vi "RT Config - Single RT Sweep.vi"(8 "error in (no error)":errorcluster, 11 "1553 Unit Test in":refnum<class "Remote Terminal.lvclass">) -> (0 "error out":errorcluster, 3 "1553 Unit Test out":refnum<class "Remote Terminal.lvclass">)   [LabVIEW 2020, in "Unit Tests.lvlib" / "Remote Terminal.lvclass"]
uses:
  Remote Terminal.lvclass
  Remote Terminal.lvclass/Remote Terminal.ctl
  Remote Terminal/TypeDefs/RT Command Config.ctl
  Frames & Messages/TypeDefs/Command Type.ctl
  Frames & Messages/TypeDefs/Command SubAddress.ctl
  Frames & Messages/TypeDefs/Command Word Count.ctl
  Frames & Messages/TypeDefs/Simplified Parameter Data Table.ctl
  Frames & Messages/TypeDefs/Scaling Information.ctl
  Remote Terminal/TypeDefs/RT Configuration.ctl
  Remote Terminal/TypeDefs/RT-RT Timeout.ctl
  Remote Terminal/TypeDefs/Mode Code 17 Sync Configuration.ctl
  Remote Terminal/TypeDefs/RT Timetag Configuration.ctl
  Remote Terminal/Remote Terminal.lvclass
  C:/Users/MattJ/Desktop/git/bci-1553-labview-api/src/1553 SubComponent/1553 SubComponent.lvclass
  1553 Session/1553 Session.lvclass
  1553 Component/1553 Component.lvclass
  <vilib>/addons/_JKI Toolkits/Caraya/classes/Test/Test.lvclass
  BCI-1553 API.lvlib
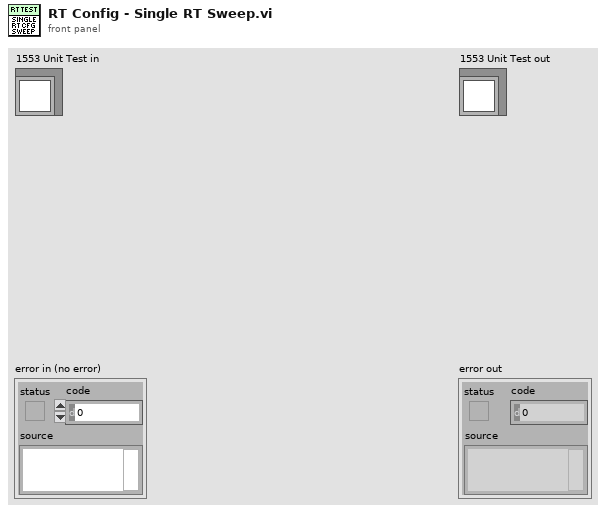
[diagram p1: front panel]
types:
  T1 = typedef "BCI-1553 API.lvlib/Simplified Parameter Data Table.ctl" = cluster{"Parameter Name":string, "Base Word":u16, "Scaling Info":T2}
  T2 = typedef "BCI-1553 API.lvlib/Scaling Information.ctl" = cluster{"Bit Offset":i32, "Bit Count":i32, "LSB Resolution":dbl, "2's Complement":bool, "Big Endian":bool, "Sign Bit":bool}
  T3 = typedef "BCI-1553 API.lvlib/Command SubAddress.ctl" = enum16{"Mode Code", "1", "2", "3", "4", "5", "6", "7", "8", "9", "10", "11", "12", "13", "14", "15", "16", "17", "18", "19", "20", "21", "22", "23", "24", "25", "26", "27", "28", "29", "30"}
  T4 = typedef "BCI-1553 API.lvlib/Command Type.ctl" = enum16{"Transmit", "Receive"}
  T5 = typedef "BCI-1553 API.lvlib/Remote Terminal.lvclass/RT Command Config.ctl" = cluster{"Command Type":T4, "SubAddress":T3, "Word Count\\Mode Code":T6, "Initial Data":u16[], "Data Fields":T1[]}
  T6 = typedef "BCI-1553 API.lvlib/Command Word Count.ctl" = enum16{"1", "2", "3", "4", "5", "6", "7", "8", "9", "10", "11", "12", "13", "14", "15", "16", "17", "18", "19", "20", "21", "22", "23", "24", "25", "26", "27", "28", "29", "30", "31", "32"}
  T7 = typedef "BCI-1553 API.lvlib/Remote Terminal.lvclass/RT Configuration.ctl" = cluster{"RT-RT Timeout":T8, "Inhibit Bus A":bool, "Inhibit Bus B":bool, "Broadcast CMD Invalid":bool, "UnDef MCs Invalid":bool, "Notice 2 Data Storage":bool, "SMCP":bool, "Temp RX Buffer":bool, "Alt BIT Enable":bool, "Auto Bus Shutdown":bool, "MC 16 SR Reset":bool, "MC 17 Sync":T9, "MC 8 Reset":bool, "Remote Terminal Timetag Config":T10}
  T8 = typedef "BCI-1553 API.lvlib/Remote Terminal.lvclass/RT-RT Timeout.ctl" = enum16{"57us", "62us", "100us", "180us"}
  T9 = typedef "BCI-1553 API.lvlib/Remote Terminal.lvclass/Mode Code 17 Sync Configuration.ctl" = enum16{"Sync if Bit 0 = 1", "Sync if Bit 0 = 0", "Sync Unconditionally"}
  T10 = typedef "BCI-1553 API.lvlib/Remote Terminal.lvclass/RT Timetag Configuration.ctl" = enum16{"Disabled", "2us", "4us", "8us", "16us", "32us", "64us"}
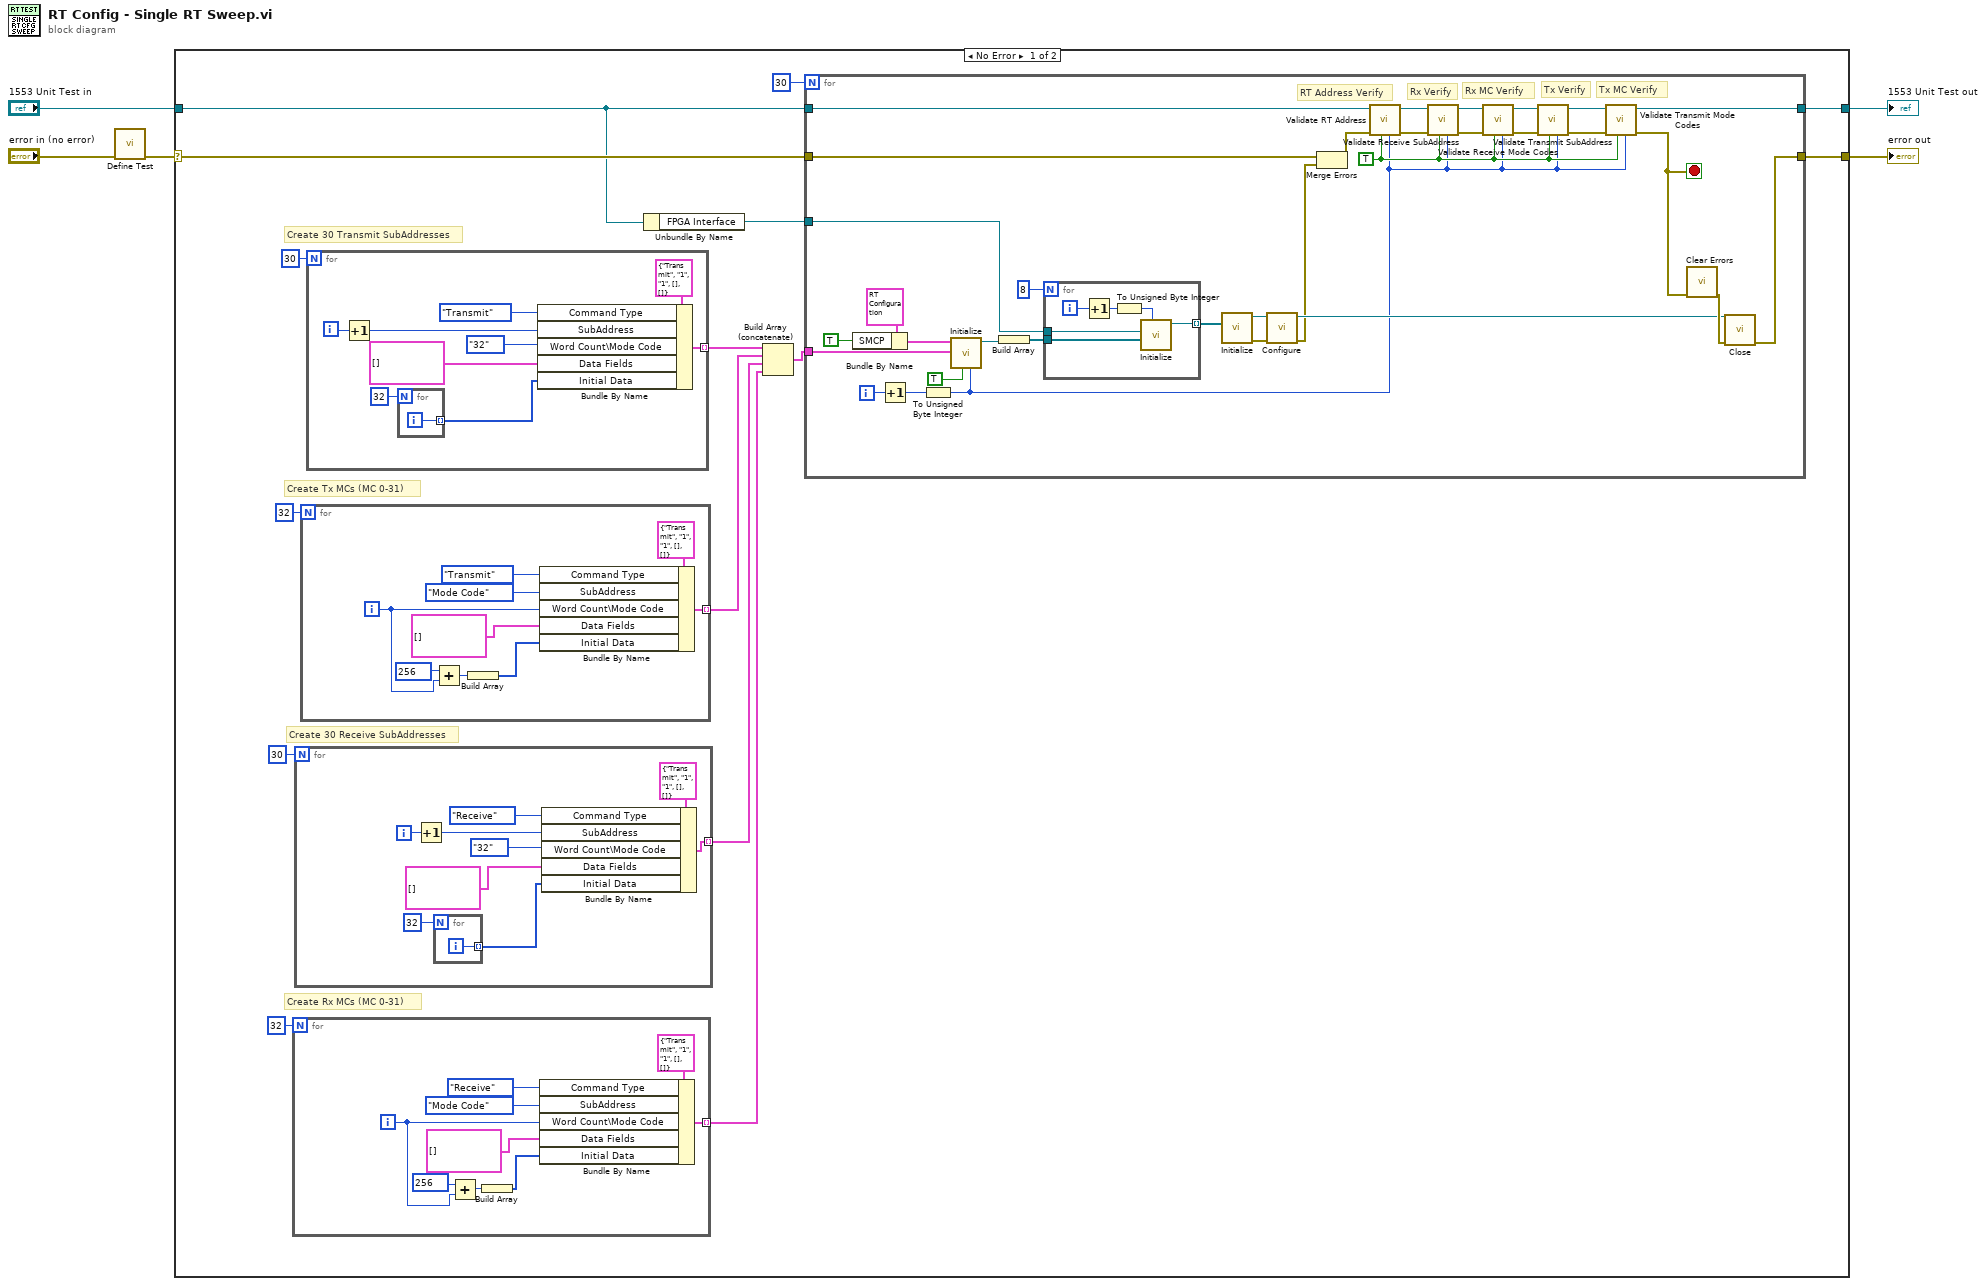
[diagram p0: block diagram]
diagram:
  n1 = call <vilib>:"Define Test.vi"("error in (no error)"="error in (no error)") -> ("error out"=w1:errorcluster)  [unwired: 9 in, 1 out]
  n2 = case shown="No Error" w1 {
    selector: w1 -> [w17 w99]
    tunnel: [w18 w99] -> w5
    tunnel: [w19 w98] -> w3
    tunnel: "1553 Unit Test in" -> [w7 w98]
    frame No Error {
      # "Create Rx MCs (MC 0-31)"
      # "Create Tx MCs (MC 0-31)"
      # "Create 30 Receive SubAddresses"
      # "Create 30 Transmit SubAddresses"
      n3 = for {
        N: 32 -> [_]
        tunnel: [w29] -> w8 mode=indexing
        i -> [w22]
        n4 = Add(x=256, y=w22) -> (x+y=w23:i32)
        n5 = Build Array(w23) -> (w25:i32[])
        n6 = Bundle By Name(cluster=T5 {"Command Type"=enum."Transmit", "SubAddress"=enum."1", "Word Count\\Mode Code"=enum."1", "Initial Data"=[], "Data Fields"=[]} ("RT Commands"), "Command Type"=Command_Type."Receive", "SubAddress"=Command_SubAddress."Mode Code", "Word Count\\Mode Code"=w22, "Data Fields"=T1[] [], "Initial Data"=w25) -> (w29:T5)
      }
      n7 = for {
        N: 30 -> [_]
        tunnel: [w47] -> w9 mode=indexing
        i -> [w42]
        n8 = Increment(x=w42) -> (x+1=w41:i32)
        n9 = for {
          N: 32 -> [_]
          tunnel: [w48] -> w43 mode=indexing
          i -> [w48]
        }
        n10 = Bundle By Name(cluster=T5 {"Command Type"=enum."Transmit", "SubAddress"=enum."1", "Word Count\\Mode Code"=enum."1", "Initial Data"=[], "Data Fields"=[]} ("RT Commands"), "Command Type"=Command_Type."Receive", "SubAddress"=w41, "Word Count\\Mode Code"=Command_Word_Count."32" ("Word Count\\Mode Code"), "Data Fields"=T1[] [], "Initial Data"=w43) -> (w47:T5)
      }
      n11 = for {
        N: 32 -> [_]
        tunnel: [w38] -> w10 mode=indexing
        i -> [w32]
        n12 = Add(x=256, y=w32) -> (x+y=w33:i32)
        n13 = Build Array(w33) -> (w31:i32[])
        n14 = Bundle By Name(cluster=T5 {"Command Type"=enum."Transmit", "SubAddress"=enum."1", "Word Count\\Mode Code"=enum."1", "Initial Data"=[], "Data Fields"=[]} ("RT Commands"), "Command Type"=Command_Type."Transmit", "SubAddress"=Command_SubAddress."Mode Code", "Word Count\\Mode Code"=w32, "Data Fields"=T1[] [], "Initial Data"=w31) -> (w38:T5)
      }
      n15 = for {
        N: 30 -> [_]
        tunnel: [w57] -> w11 mode=indexing
        i -> [w52]
        n16 = Increment(x=w52) -> (x+1=w51:i32)
        n17 = for {
          N: 32 -> [_]
          tunnel: [w58] -> w53 mode=indexing
          i -> [w58]
        }
        n18 = Bundle By Name(cluster=T5 {"Command Type"=enum."Transmit", "SubAddress"=enum."1", "Word Count\\Mode Code"=enum."1", "Initial Data"=[], "Data Fields"=[]} ("RT Commands"), "Command Type"=Command_Type."Transmit", "SubAddress"=w51, "Word Count\\Mode Code"=Command_Word_Count."32" ("Word Count\\Mode Code"), "Data Fields"=T1[] [], "Initial Data"=w53) -> (w57:T5)
      }
      n19 = Unbundle By Name(w7) -> ("FPGA Interface"=w6:refnum<class "FPGA Interface.lvclass">)
      n20 = Build Array (concatenate)(w11, w10, w9, w8) -> (w16:T5[])
      n21 = for {
        N: 30 -> [_]
        tunnel: [w69] -> w18
        tunnel: w17 -> [w75]
        tunnel: w7 -> [w79]
        tunnel: [w61] -> w19
        tunnel: w16 -> [w70]
        tunnel: w6 -> [w72]
        i -> [w86]
        stop <- w62 stop-if-true
        w60 = TRUE ("RT 1?")
        # "Tx MC Verify"
        # "Rx MC Verify"
        # "Tx Verify"
        # "Rx Verify"
        # "RT Address Verify"
        n22 = Bundle By Name(cluster=T7 {"RT-RT Timeout"=enum."57us", "Inhibit Bus A"=FALSE, "Inhibit Bus B"=FALSE, "Broadcast CMD Invalid"=FALSE, "UnDef MCs Invalid"=FALSE, "Notice 2 Data Storage"=FALSE, "SMCP"=FALSE, "Temp RX Buffer"=FALSE, "Alt BIT Enable"=FALSE, "Auto Bus Shutdown"=FALSE, "MC 16 SR Reset"=FALSE, "MC 17 Sync"=enum."Sync if Bit 0 = 1", "MC 8 Reset"=FALSE, "Remote Terminal Timetag Config"=enum."Disabled"} ("RT Configuration"), "SMCP"=TRUE) -> (w90:T7)
        n23 = Increment(x=w86) -> (x+1=w87:i32)
        n24 = To Unsigned Byte Integer(number=w87) -> (unsigned 8bit integer=w59:u8)
        n25 = call "Initialize.vi"("Terminal Address"=w59, "RT 1?"=TRUE, "RT Commands"=w70, "RT Configuration"=w90) -> ("Remote Terminal out"=w83:refnum<class "Remote Terminal.lvclass">)  [unwired: 6 in, 1 out]
        n26 = Build Array(w83) -> (w85:refnum<class "Remote Terminal.lvclass">[])
        n27 = for {
          N: 8 -> [_]
          tunnel: [w95] -> w82 mode=indexing
          tunnel: w85 -> [w94]
          tunnel: w72 -> [w93]
          i -> [w97]
          n28 = Increment(x=w97) -> (x+1=w92:i32)
          n29 = To Unsigned Byte Integer(number=w92) -> (unsigned 8bit integer=w96:u8)
          n30 = call "Initialize.vi"("Component ID (1-8)"=w96, "SubComponents"=w94, "FPGA Interface"=w93) -> ("1553 Component out"=w95:refnum<class "1553 Component.lvclass">)  [unwired: 7 in, 1 out]
        }
        n31 = call "Initialize.vi"("Components"=w82) -> ("error out"=w80:errorcluster, "1553 Board out"=w81:refnum<class "1553 Session.lvclass">)  [unwired: 9 in]
        n32 = call-dynamic "Configure.vi"("error in (no error)"=w80, "1553 Board in"=w81) -> ("error out"=w71:errorcluster, "1553 Board out"=w76:refnum<class "1553 Session.lvclass">)  [unwired: 8 in]
        n33 = Merge Errors(w75, w71) -> (w78:errorcluster)
        n34 = call "Validate RT Address.vi"("RT Address (0-30)"=w59, "RT 1?"=w60, "error in (no error)"=w78, "Remote Terminal in"=w79) -> ("error out"=w73:errorcluster, "Remote Terminal out"=w74:refnum<class "Remote Terminal.lvclass">)  [unwired: 6 in]
        n35 = call "Validate Receive SubAddress.vi"("RT Address (0-30)"=w59, "RT 1?"=w60, "error in (no error)"=w73, "1553 Unit Test in"=w74) -> ("error out"=w66:errorcluster, "1553 Unit Test out"=w68:refnum<class "Remote Terminal.lvclass">)  [unwired: 6 in]
        n36 = call "Validate Receive Mode Codes.vi"("RT Address (0-30)"=w59, "RT 1?"=w60, "error in (no error)"=w66, "1553 Unit Test in"=w68) -> ("error out"=w65:errorcluster, "1553 Unit Test out"=w67:refnum<class "Remote Terminal.lvclass">)  [unwired: 6 in]
        n37 = call "Validate Transmit SubAddress.vi"("RT Address (0-30)"=w59, "RT 1?"=w60, "error in (no error)"=w65, "1553 Unit Test in"=w67) -> ("error out"=w63:errorcluster, "1553 Unit Test out"=w64:refnum<class "Remote Terminal.lvclass">)  [unwired: 6 in]
        n38 = call "Validate Transmit Mode Codes.vi"("RT Address (0-30)"=w59, "RT 1?"=w60, "error in (no error)"=w63, "1553 Unit Test in"=w64) -> ("error out"=w62:errorcluster, "1553 Unit Test out"=w61:refnum<class "Remote Terminal.lvclass">)  [unwired: 6 in]
        n39 = call <vilib>:"Clear Errors.vi"("error in (no error)"=w62) -> ("error out"=w77:errorcluster)  [unwired: 5 in, 1 out]
        n40 = call-dynamic "Close.vi"("error in (no error)"=w77, "1553 Board in"=w76) -> ("error out"=w69:errorcluster)  [unwired: 9 in]
      }
    }
    frame Error {
    }
  }
  "error out" <- w5
  "1553 Unit Test out" <- w3
